vi "User Test Info.vi"(0 "CONFIG IN":T1, 11 "Error IN":errorcluster) -> (4 "CONFIG OUT":T1, 8 "Cancelled?":bool=TRUE, 15 "Error OUT":errorcluster)   [LabVIEW 2012]
panel:
  in  "Cancel Button":bool
  in  "OK Button":bool
  in  "Alternate Email (Optional)":string
  in  "Last Name":string
  in  "First Name":string
  in  "Test Name":string
  in  "Test Description":string
  # "(first.last@ecolab.com)"
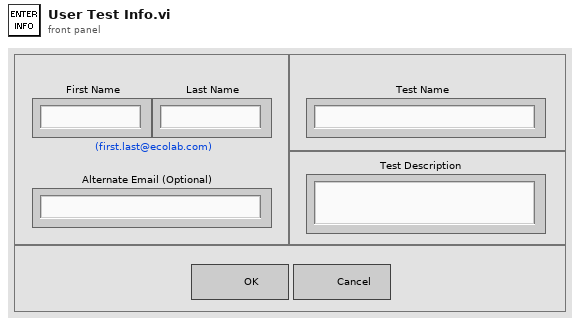
[diagram p1: front panel]
types:
  T1 = cluster{"First Name":string, "Last Name":string, "Alternate Email":string, "Test Name":string, "Test Description":string}
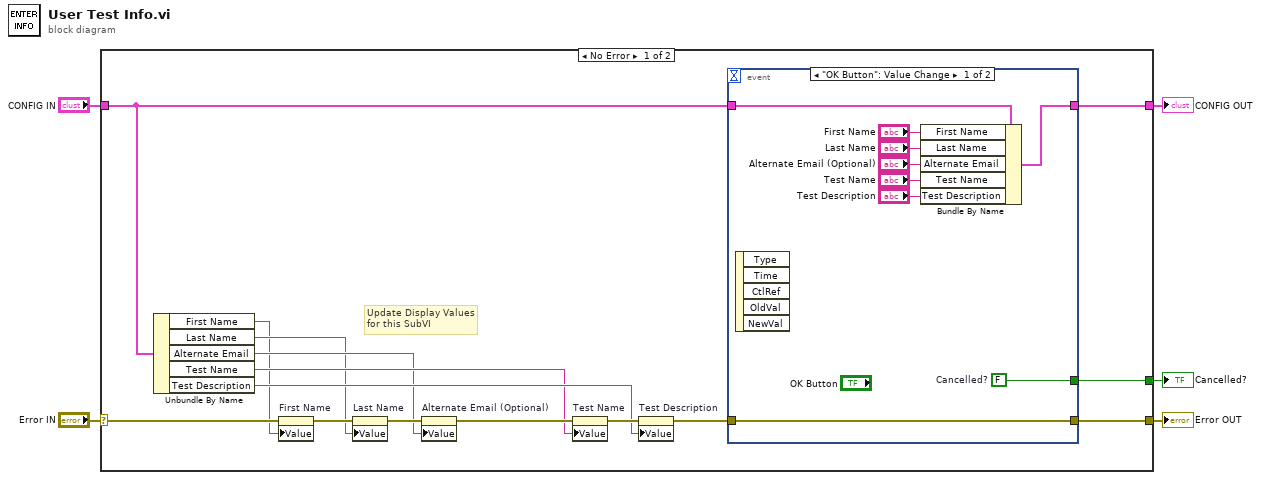
[diagram p0: block diagram]
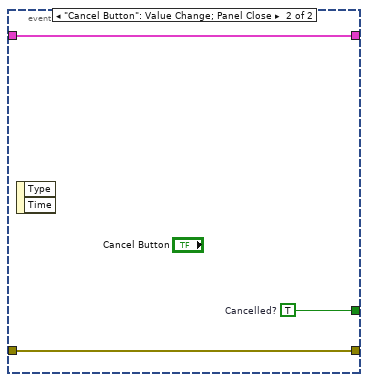
[diagram p2: hidden frame]
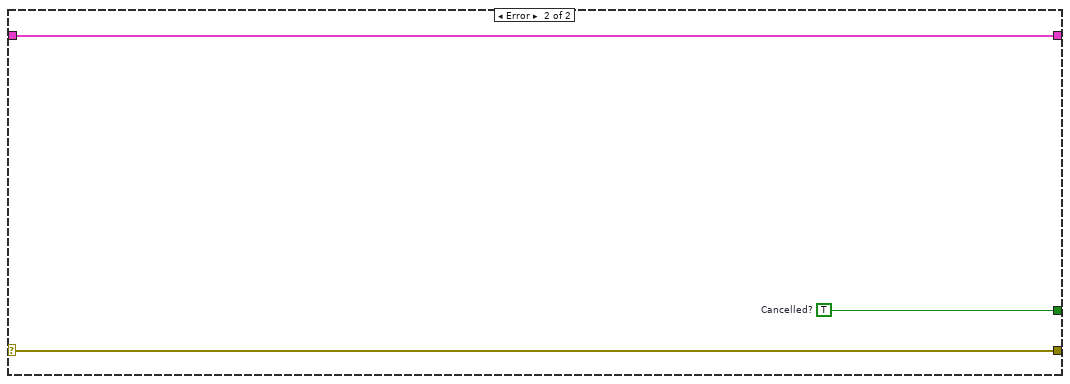
[diagram p3: hidden frame]
diagram:
  n1 = case shown="No Error" "Error IN" {
    selector: "Error IN" -> [w11 w34]
    tunnel: "CONFIG IN" -> [w17 w35]
    tunnel: [w20 w35] -> w4
    tunnel: [w18 w34] -> w2
    tunnel: [w19 w33] -> w1
    frame No Error {
      # "Update Display Values\nfor this SubVI"
      n2 = Unbundle By Name(w17) -> ("First Name"=w6:string, "Last Name"=w7:string, "Alternate Email"=w8:string, "Test Name"=w9:string, "Test Description"=w10:string)
      n3 = property on="First Name" class="Str"(error in=w11, "Value"=w6) -> (error out=w16:errorcluster)  [unwired: 1 in, 1 out]
      n4 = property on="Last Name" class="Str"(error in=w16, "Value"=w7) -> (error out=w15:errorcluster)  [unwired: 1 in, 1 out]
      n5 = property on="Alternate Email (Optional)" class="Str"(error in=w15, "Value"=w8) -> (error out=w14:errorcluster)  [unwired: 1 in, 1 out]
      n6 = property on="Test Name" class="Str"(error in=w14, "Value"=w9) -> (error out=w13:errorcluster)  [unwired: 1 in, 1 out]
      n7 = property on="Test Description" class="Str"(error in=w13, "Value"=w10) -> (error out=w12:errorcluster)  [unwired: 1 in, 1 out]
      n8 = event shown="[0] \"OK Button\": Value Change" {
        selector: _ -> [_ _]
        dyn-events: _ -> [_ _]
        timeout: _ -> [_ _]
        tunnel: w17 -> [w28 w32]
        tunnel: [w27 w32] -> w20
        tunnel: [w21 w31] -> w19
        tunnel: w12 -> [w22 w30]
        tunnel: [w22 w30] -> w18
        event "OK Button": Value Change {
          w21 = FALSE  # Cancelled?
          n9 = event-data() -> ()  [unwired: 1 in, 5 out]
          n10 = Bundle By Name(cluster=w28, "First Name"="First Name", "Last Name"="Last Name", "Alternate Email"="Alternate Email (Optional)", "Test Name"="Test Name", "Test Description"="Test Description") -> (w27:T1)
        }
        event "Cancel Button": Value Change; Panel Close {
          w31 = TRUE  # Cancelled?
          n11 = event-data() -> ()  [unwired: 1 in, 2 out]
        }
      }
    }
    frame Error {
      w33 = TRUE  # Cancelled?
    }
  }
  "CONFIG OUT" <- w4
  "Error OUT" <- w2
  "Cancelled?" <- w1
